vi "Enable Math.vi"(8 "error in":errorcluster, 10 "Enable (F: Disable)":bool, 11 "VISA resource name":refnum<visa-resource-name>) -> (0 "error out":errorcluster, 3 "VISA resource name out":refnum<visa-resource-name>)   [LabVIEW 2013, in "DmmPwr Simulator.lvlib"]
doc: "Enables or disables the calculations."
uses:
  <instrlib>/DmmPwr Simulator/DmmPwr Simulator.lvlib
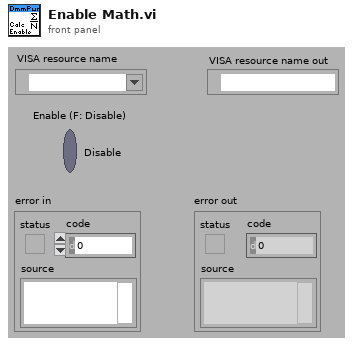
[diagram p1: front panel]
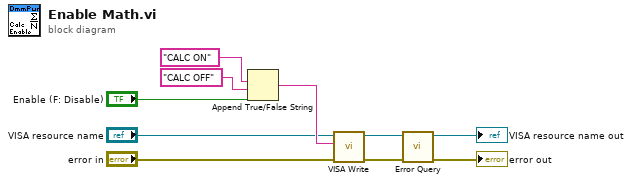
[diagram p0: block diagram]
diagram:
  n1 = Append True/False String(1:"Enable (F: Disable)", 2:"CALC OFF", 3:"CALC ON") -> (0:w6:string)  [unwired: 1 out]
  n2 = call <instrlib>:"VISA Write.vi"("error in"="error in", "write buffer"=w6, "VISA resource name"="VISA resource name") -> ("error out"=w7:errorcluster, "VISA resource name out"=w8:refnum<visa-resource-name>)  [unwired: 6 in, 1 out]
  n3 = call <instrlib>:"Error Query.vi"("error in (no error)"=w7, "VISA resource name"=w8) -> ("error out"=→"error out":errorcluster, "VISA resource name out"=→"VISA resource name out":refnum<visa-resource-name>)  [unwired: 6 in, 2 out]
